vi "CalibBoard.vi"() -> ()   [LabVIEW 2014]
uses:
  <vilib>/userdefined/High Color/IMAQdx.ctl
  <vilib>/vision/Image Controls.llb/IMAQ Image.ctl
  Ctrl/CalibBoardAction.ctl
  <vilib>/Utility/miscctls.llb/LVPositionTypeDef.ctl
  Ctrl/ColorImg.ctl
  Control/RobotActionMode.ctl
  Global/PanelSetting.vi
  <vilib>/vision/driver/NI_Vision_Acquisition_Software.lvlib
panel:
  in  "SelectCalib":bool caption="點位校正功能開啟"
  out "UpCamTool 2":cluster{"CP-J1-X":sgl, "CP-J2-Y":sgl}={"CP-J1-X"=-0.14151, "CP-J2-Y"=-65.0295} caption="相機中心" {"CP-J2-Y" format="%.3g"; "CP-J1-X" format="%.3g"}
  out "UpCamTool":refnum<vi>
  in  "Session In":T1
  in  "Btn_BoardSave":bool
  in  "file path (use dialog)":path
  out "ActQ":refnum<queue>
  in  "CalibPts":cluster{"X":dbl, "Y":dbl, "Z":dbl, "U":dbl}[](array[cluster])
  out "BoardPts":cluster{dbl, dbl}[][](array[cluster])
  out "CalibPoint":cluster{dbl, dbl}[](array[cluster])
  out "Current PositionRef":refnum<vi>
  in  "Current Position":T2 caption="當前點位坐標" {"CP-J6-W" format="%.3g"; "CP-J5-V" format="%.3g"; "CP-J4-U" format="%.3g"; "CP-J3_Z" format="%.3g"; "CP-J2-Y" format="%.3g"; "CP-J1-X" format="%.3g"}
  in  "Image":T3
  out "Btn_ExistRef":refnum<vi>
  in  "Btn_Exist":bool=TRUE
  in  "Tab Control":enum32{"Set", "Data"}(tab)
  out "CirclesResult":T4(array[cluster]) caption="圓結果"
  in  "SetStartPoint":bool
  in  "PointArray":cluster{"X":i32, "Y":i32} caption="標準板陣列"
  in  "PointsDis":cluster{"DeltaX":dbl, "DeltaY":dbl} caption="點距離(mm)"
  in  "StartPoint":cluster{"X":dbl, "Y":dbl, "Z":dbl, "U":dbl} caption="起始點位"
  in  "StartCalib":bool
  in  "CalibBoardImg":T3(plugin-control)
  in  "Clu_BoardCircleParameter":T5={"Extraction Mode"=enum."Normal", "Edge Threshold"=40, "Edge Filter Size"=enum."Normal"} caption="搜尋參數"
  in  "Btn_SetROI":bool
  in  "Btn_BoardDetect":bool
  in  "Btn_BoardSnap":bool
  in  "Circle Descriptor":cluster{"Min Radius":dbl, "Max Radius":dbl}={"Min Radius"=30.0, "Max Radius"=100.0} caption="圓半徑"
  in  "ROI":T6
  out "Numbers":i32
  in  "Index":i32
  in  "CalibBoardData":string[][](table)
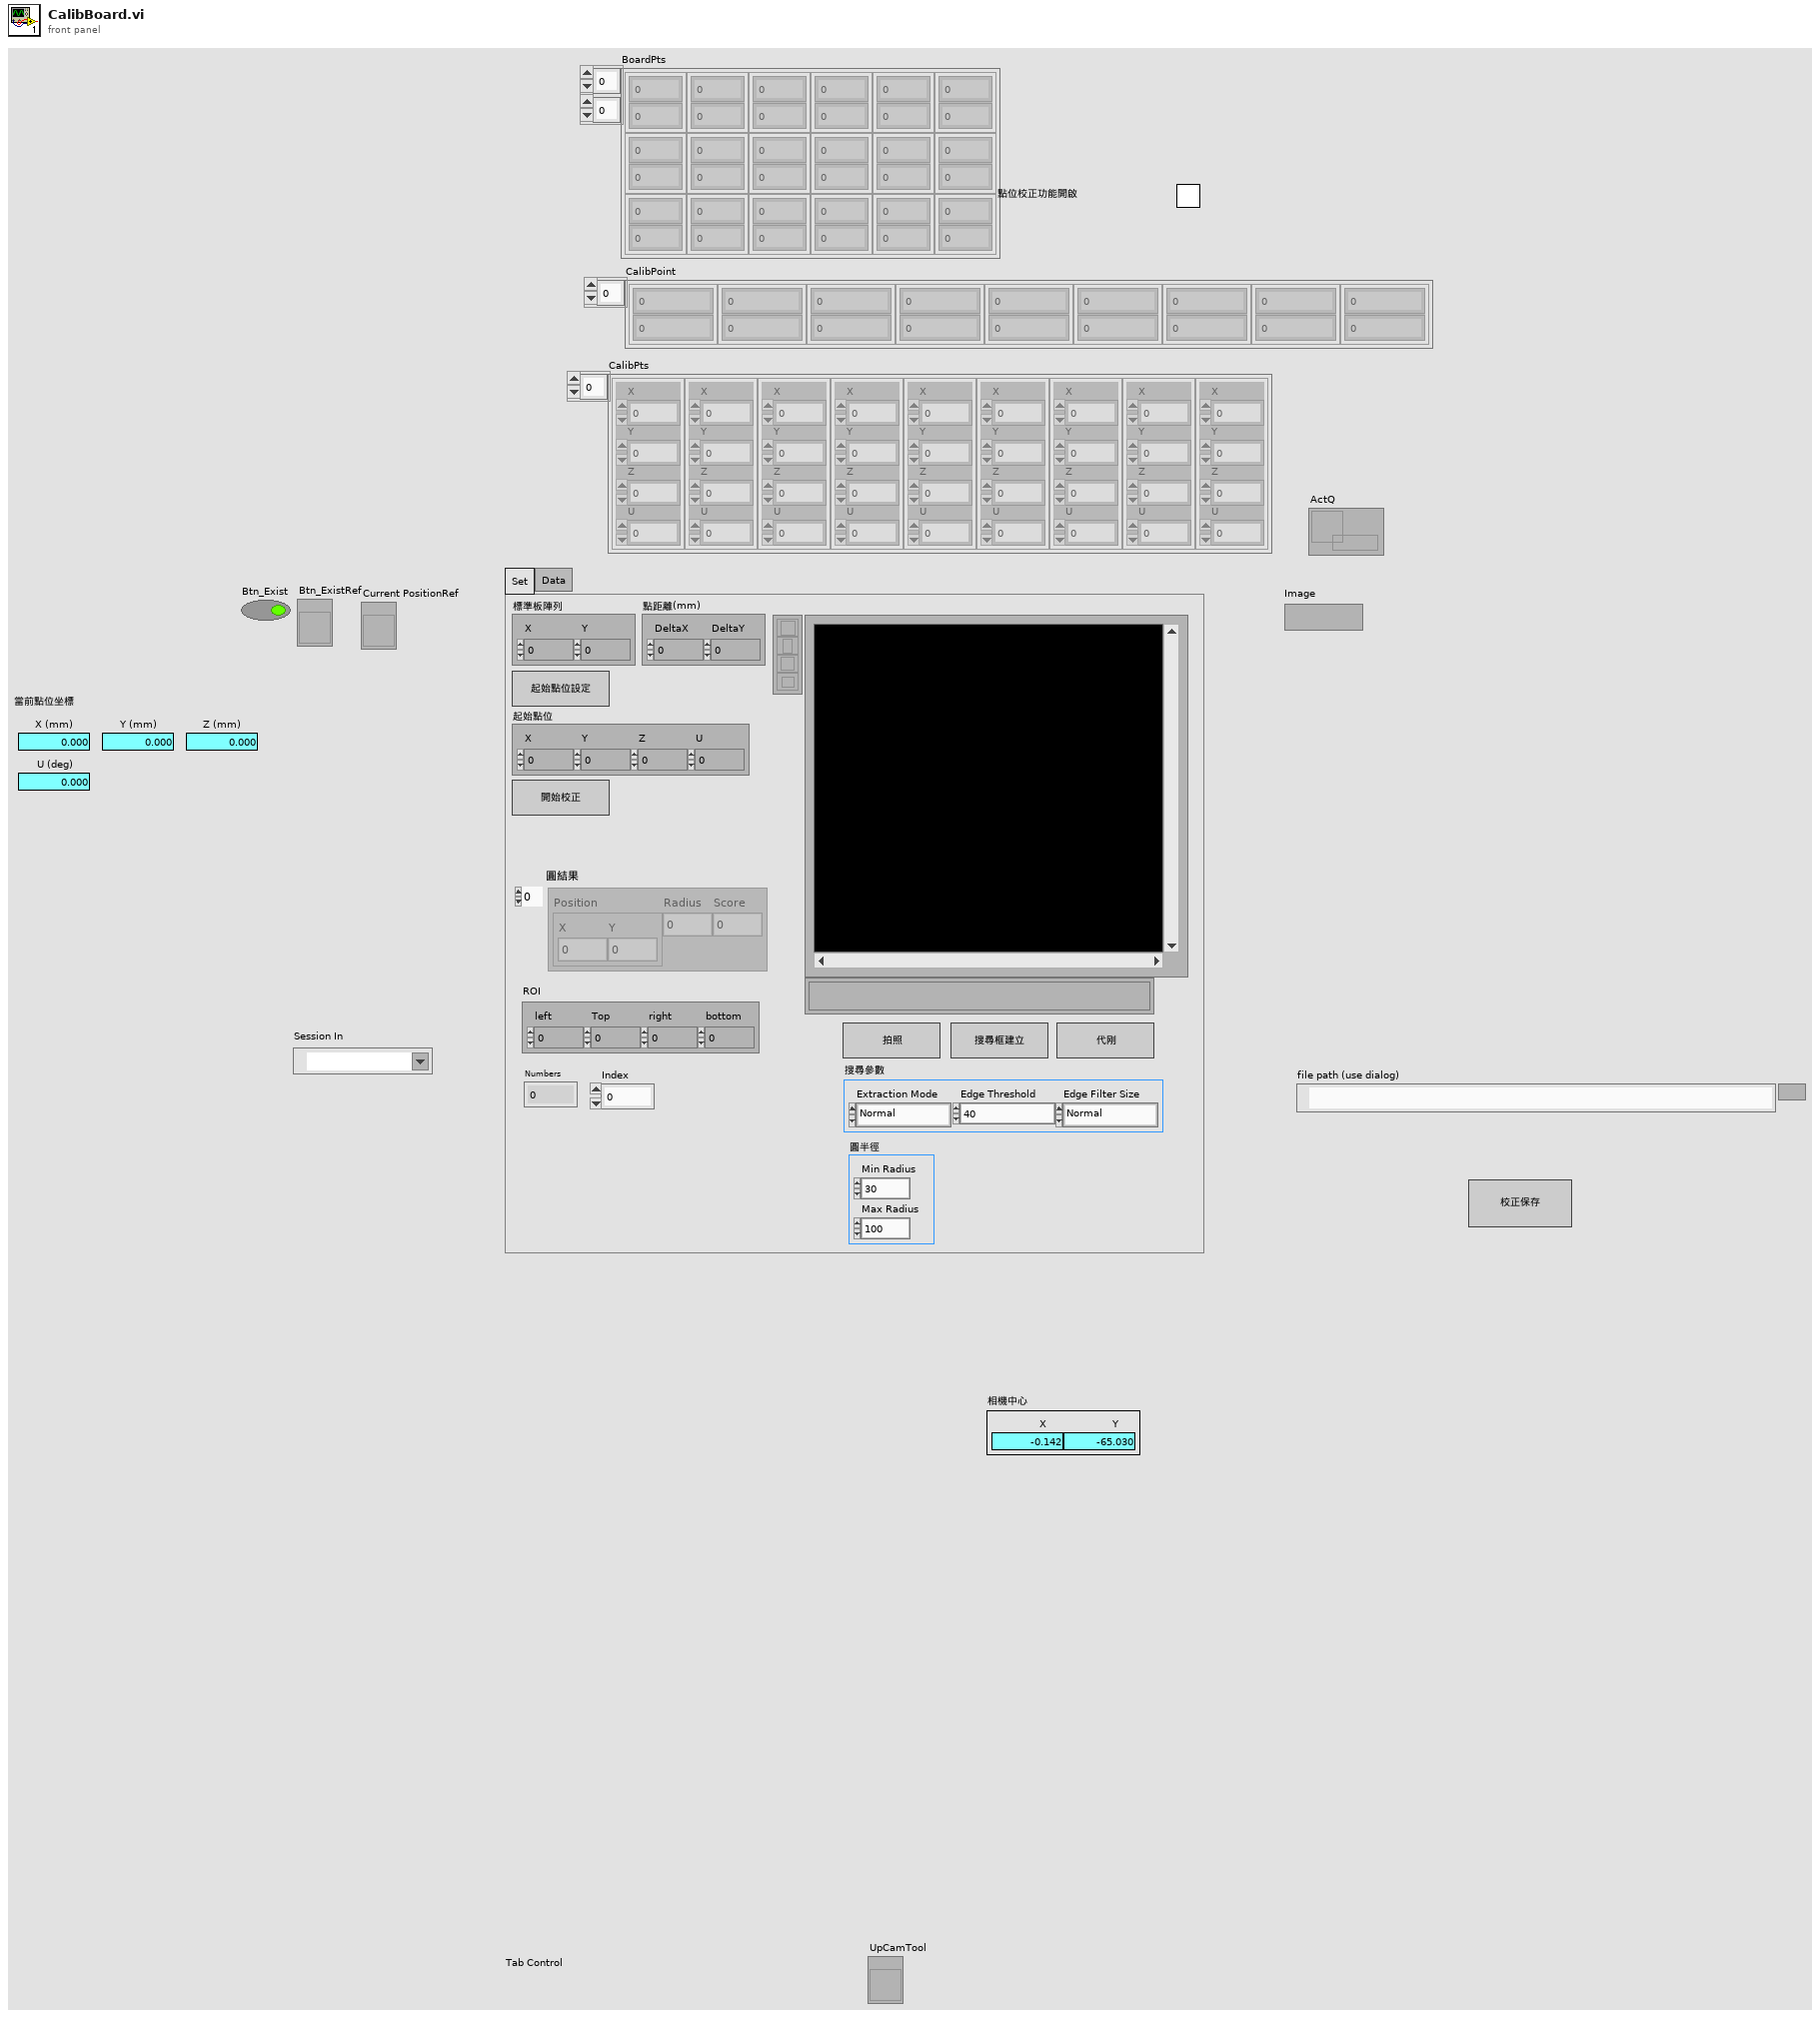
[diagram p1: front panel]
types:
  T1 = typedef "IMAQdx.ctl" = refnum<k21>
  T2 = cluster{"CP-J1-X":sgl, "CP-J2-Y":sgl, "CP-J3_Z":sgl, "CP-J4-U":sgl, "CP-J5-V":sgl, "CP-J6-W":sgl}
  T3 = typedef "IMAQ Image.ctl" = refnum<image>
  T4 = cluster{"Position":cluster{"X":sgl, "Y":sgl}, "Radius":dbl, "Score":dbl}[]
  T5 = cluster{"Extraction Mode":enum16{"Normal", "Uniform Regions"}, "Edge Threshold":i32, "Edge Filter Size":enum16{"Fine", "Normal"}}
  T6 = cluster{"left":i32, "Top":i32, "right":i32, "bottom":i32}
  T7 = enum16{"initialref", "save", "load", "UpDataToUI", "write", "read"}
  T8 = typedef "CalibBoardAction.ctl" = enum16{"CalibBoard", "Snap", "BoardCircleDectect", "CaculateOffset", "Exit"}
  T9 = typedef "RobotActionMode.ctl" = cluster{"PM_1":i32, "PM_2":i32}
  T10 = typedef "ColorImg.ctl" = enum16{"CBSource", "CBShow", "CBToProcess"}
  T11 = cluster{"Curve Parameters":cluster{"Extraction Mode":enum16{"Normal", "Uniform Regions"}, "Edge Threshold":i32, "Edge Filter Size":enum16{"Fine", "Normal"}, "Min Length":i32, "Row Search Step Size":i32, "Col Search Step Size":i32, "Max Endpoint Gap":i32, "Closed":bool, "Subpixel":bool}, "Circle Descriptor":cluster{"Min Radius":dbl, "Max Radius":dbl}, "Match Options":cluster{"Rotation":bool, "Scale":bool, "Occlusion":bool, "Range Settings":cluster{"Match Constraints":enum16{"Rotation Angle (degrees)", "Scale Factor (%)", "Occlusion (%)"}, "Min":dbl, "Max":dbl}[]}, "Minimum match score":dbl, "SetCircleNum":i32}
  T12 = typedef "LVPositionTypeDef.ctl" = cluster{"Left":i32, "Top":i32}
  T13 = cluster{"PointArray":refnum<vi>, "PointsDis":refnum<vi>, "StartPoint":refnum<vi>, "ROI":refnum<vi>, "Clu_BoardCircleParameter":refnum<vi>, "Circle Descriptor":refnum<vi>, "BoardPts":refnum<vi>, "CalibPoint":refnum<vi>, "CalibPts":refnum<vi>, "SelectCalib":refnum<vi>}
  T14 = cluster{"Global Rectangle":i32[], "Contours":cluster{"Contour Type":u32, "ROI Type":u32, "Points":i32[]}[]}
  T15 = typedef "IMAQ Rectangle" = cluster{"Left":i32, "Top":i32, "Right":i32, "Bottom":i32, "Rotation":dbl}
  T16 = cluster{"Left":i32, "Top":i32, "Right":i32, "Bottom":i32}
  T17 = cluster{"CP-J1-X":sgl, "CP-J2-Y":sgl, "CP-J3_Z":sgl, "CP-J4-U":sgl}
  T18 = cluster{"left":i32, "Top":i32, "right":i32, "bottom":i32, dbl}
  T19 = typedef "ROI Descriptor" = cluster{"Global Rectangle":i32[], "Contours":cluster{"ID":enum32{"External", "Internal"}, "Type":u32, "Coordinates":i32[]}[]}
  T20 = cluster{"Position":cluster{"X":sgl, "Y":sgl}, "Radius":dbl, "Score":dbl}
  T21 = cluster{"[0]":sgl, "[1]":sgl, "[2]":sgl, "[3]":sgl}
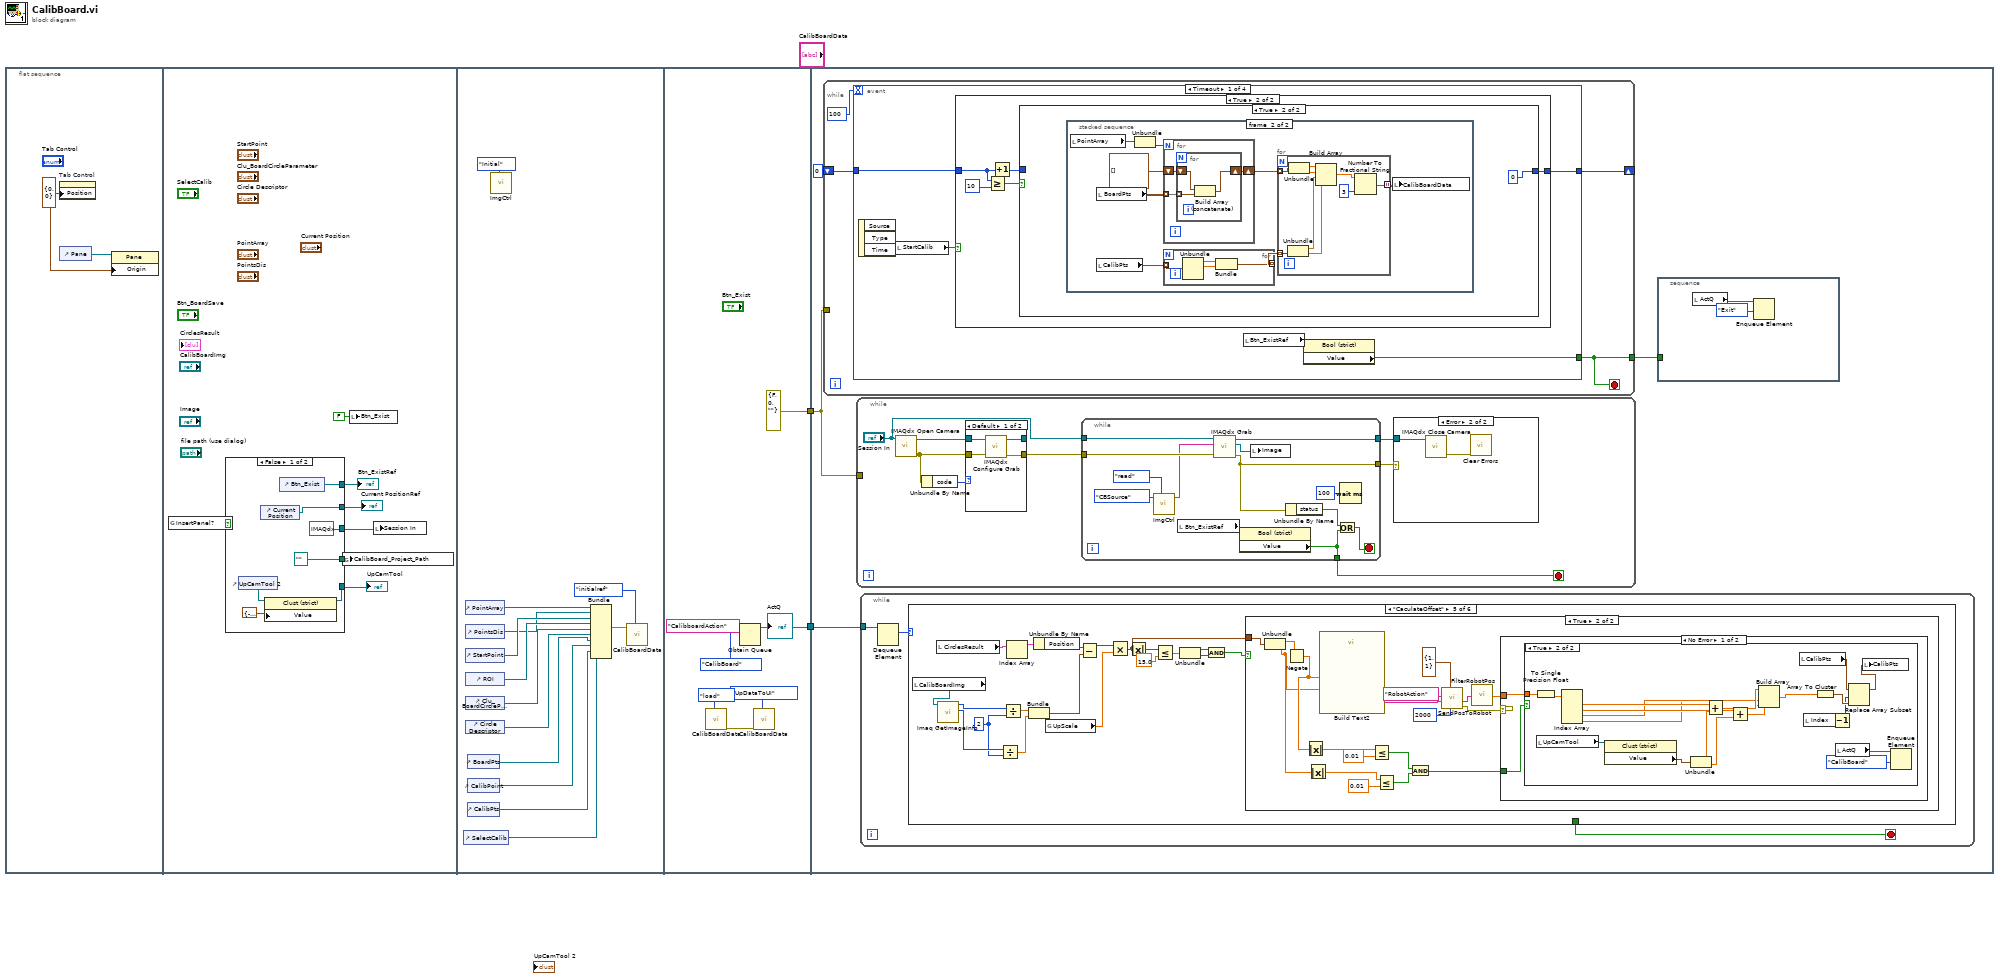
[diagram p0: block diagram]
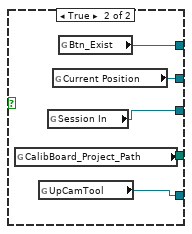
[diagram p2: hidden frame]
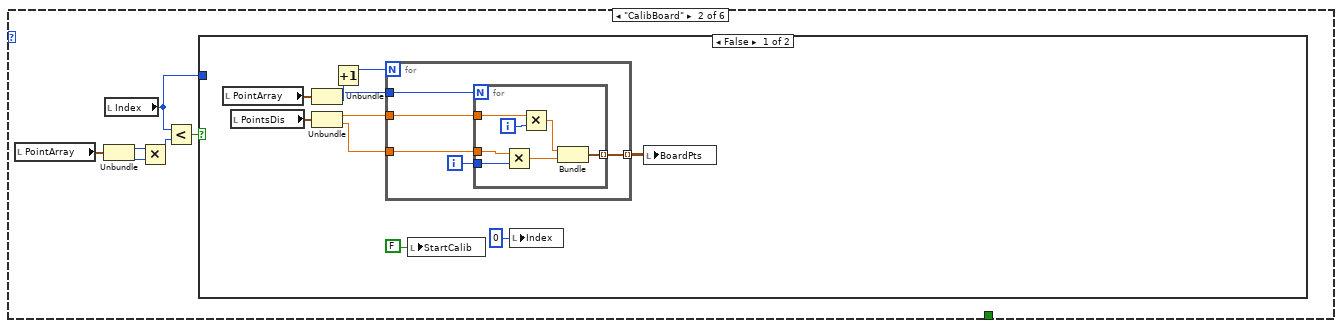
[diagram p4: hidden frame]
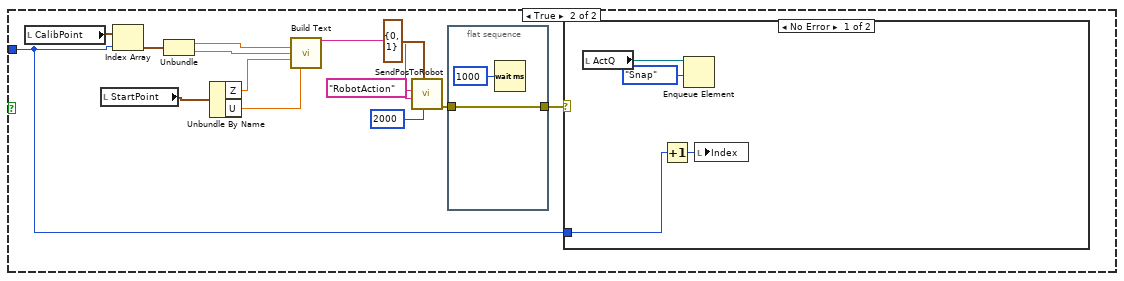
[diagram p5: hidden frame]
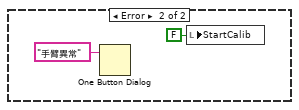
[diagram p6: hidden frame]
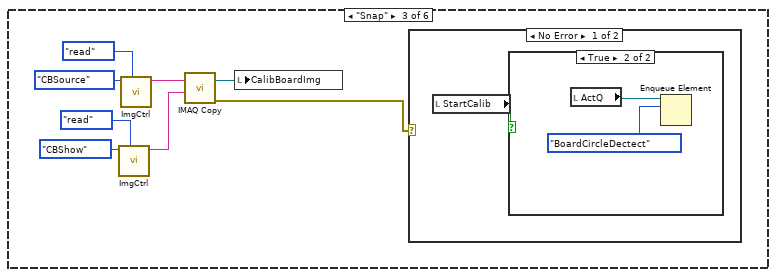
[diagram p7: hidden frame]
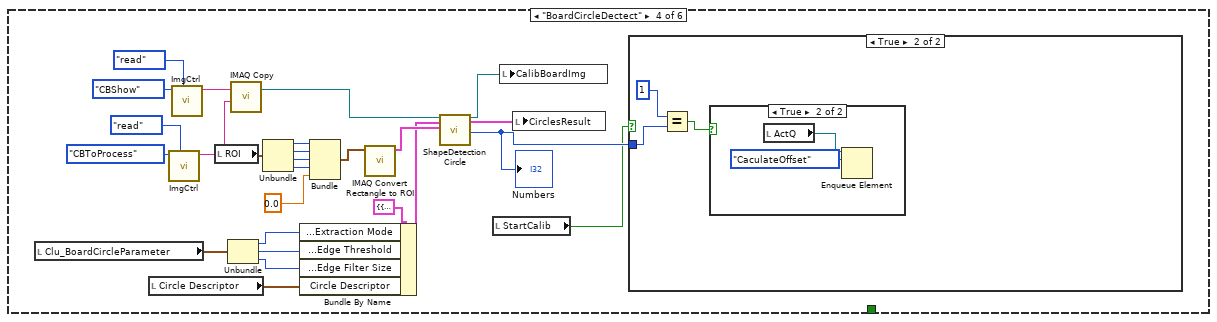
[diagram p10: hidden frame]
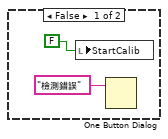
[diagram p12: hidden frame]
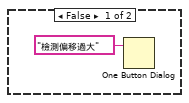
[diagram p13: hidden frame]
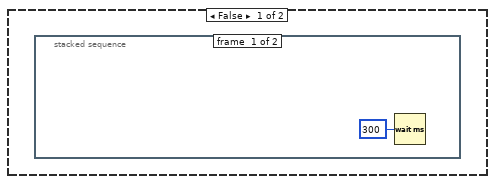
[diagram p14: hidden frame]
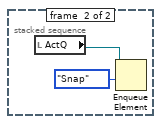
[diagram p15: hidden frame]
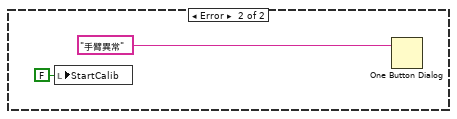
[diagram p16: hidden frame]
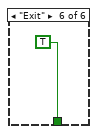
[diagram p17: hidden frame]
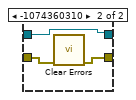
[diagram p18: hidden frame]
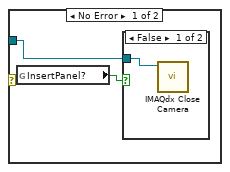
[diagram p19: hidden frame]
diagram:
  n1 = flat-sequence {
    tunnel: [errorcluster {"status"=FALSE, "code"=0, "source"=""} ("error constant")] -> w2
    tunnel: [w40] -> w1
    tunnel: w2 -> [w47]
    tunnel: w1 -> [w46]
    frame #0 {
      w3 = T12 {"Left"=0, "Top"=0} ("Position")
      n2 = property on="Tab Control" class="TabCtl (strict)"("Position"=w3) -> ()  [unwired: 2 in, 2 out]
      n3 = control-ref of="Pane"() -> (w4:refnum<vi>)
      n4 = property class="Pane"(reference=w4, "Origin"=w3) -> ()  [unwired: 1 in, 2 out]
    }
    frame #1 {
      n5 = global read "PanelSetting.vi" "InsertPanel?"() -> (w11:bool)
      n6 = case shown="False" w11 {
        tunnel: [w18 w23] -> w10
        tunnel: [w17 w22] -> w9
        tunnel: [T1 refnum ("Session In") w21] -> w8
        tunnel: [path "" ("Project_Path") w20] -> w6
        tunnel: [w12 w19] -> w5
        frame False {
          n7 = control-ref of="UpCamTool 2"() -> (w14:refnum<vi>)
          n8 = control-ref of="Current Position"() -> (w17:refnum<vi>)
          n9 = property class="Clust (strict)"(reference=w14, "Value"=cluster{"CP-J1-X":sgl, "CP-J2-Y":sgl} {"CP-J1-X"=-0.142, "CP-J2-Y"=-65.03}) -> (reference out=w12:refnum<vi>)  [unwired: 1 in, 1 out]
          n10 = control-ref of="Btn_Exist"() -> (w18:refnum<vi>)
        }
        frame True {
          n11 = global read "PanelSetting.vi" "CalibBoard_Project_Path"() -> (w20:path)
          n12 = global read "PanelSetting.vi" "UpCamTool"() -> (w19:refnum<vi>)
          n13 = global read "PanelSetting.vi" "Session In"() -> (w21:T1)
          n14 = global read "PanelSetting.vi" "Current Position"() -> (w22:refnum<vi>)
          n15 = global read "PanelSetting.vi" "Btn_Exist"() -> (w23:refnum<vi>)
        }
      }
      "Btn_ExistRef" <- w10
      "Current PositionRef" <- w9
      "UpCamTool" <- w5
      n16 = global write "PanelSetting.vi" "CalibBoard_Project_Path"(w6) -> ()
      n17 = local write "Btn_Exist"(FALSE ("Btn_Exist")) -> ()
      n18 = local write "Session In"(w8) -> ()
    }
    frame #2 {
      n19 = control-ref of="SelectCalib"() -> (w24:refnum<vi>)
      n20 = control-ref of="PointArray"() -> (w27:refnum<vi>)
      n21 = control-ref of="PointsDis"() -> (w28:refnum<vi>)
      n22 = control-ref of="StartPoint"() -> (w29:refnum<vi>)
      n23 = control-ref of="ROI"() -> (w30:refnum<vi>)
      n24 = control-ref of="Clu_BoardCircleParameter"() -> (w31:refnum<vi>)
      n25 = control-ref of="Circle Descriptor"() -> (w32:refnum<vi>)
      n26 = control-ref of="BoardPts"() -> (w33:refnum<vi>)
      n27 = control-ref of="CalibPoint"() -> (w34:refnum<vi>)
      n28 = control-ref of="CalibPts"() -> (w35:refnum<vi>)
      n29 = call "ImgCtrl.vi"("Action"=enum16{"Initial", "read", "release"}."Initial") -> ()  [unwired: 9 in, 2 out]
      n30 = Bundle("PointArray"=w27, "PointsDis"=w28, "StartPoint"=w29, "ROI"=w30, "Clu_BoardCircleParameter"=w31, "Circle Descriptor"=w32, "BoardPts"=w33, "CalibPoint"=w34, "CalibPts"=w35, "SelectCalib"=w24) -> (w26:T13)  [unwired: 1 in]
      n31 = call "CalibBoardData.vi"("Enum"=T7."initialref", "RefIn"=w26) -> ()  [unwired: 8 in, 2 out]
    }
    frame #3 {
      n32 = call "CalibBoardData.vi"("Enum"=T7."load") -> ("error out"=w37:errorcluster)  [unwired: 9 in, 1 out]
      n33 = Obtain Queue(name (unnamed)="CalibboardAction", element data type=CalibBoardAction."CalibBoard") -> (queue out=w40:refnum<queue>)  [unwired: 3 in, 2 out]
      "ActQ" <- w40
      n34 = call "CalibBoardData.vi"("Enum"=T7."UpDataToUI", "error in"=w37) -> ()  [unwired: 8 in, 2 out]
    }
    frame #4 {
      n35 = while {
        tunnel: w47 -> [_]
        tunnel: [w248] -> w45
        shift-right: [w246] -> _
        shift-left: 0 -> [w247]
        stop <- w248 stop-if-true
        n36 = event shown="[0] Timeout" {
          selector: _ -> [_ _ _ _]
          dyn-events: _ -> [_ _ _ _]
          timeout: 100 -> [_ _ _ _]
          tunnel: [w254 _ _ _] -> w248
          tunnel: w247 -> [w251 _ _ _]
          tunnel: [w250 _ _ _] -> w246
          event Timeout {
            n37 = event-data() -> ()  [unwired: 1 in, 3 out]
            n38 = local read "StartCalib"() -> (w252:bool)
            n39 = case shown="True" w252 {
              tunnel: w251 -> [w255 w257]
              tunnel: [w255 w258] -> w250
              frame False {
              }
              frame True {
                n40 = Greater Or Equal?(x=w257, y=10) -> (x >= y?=w259:bool)
                n41 = Increment(x=w257) -> (x+1=w256:i32)
                n42 = case shown="True" w259 {
                  tunnel: [w261 0] -> w258
                  tunnel: w256 -> [w261 _]
                  frame False {
                  }
                  frame True {
                    n43 = stacked-sequence {
                      frame #0 {
                        n44 = local read "PointArray"() -> (w267:cluster{"X":i32, "Y":i32})
                        n45 = Unbundle(w267) -> ("X"=w265:i32, "Y"=w266:i32)
                        n46 = Multiply(x=w265, y=w266) -> (x*y=w264:i32)
                        n47 = for {
                          N: w264 -> [_]
                          tunnel: [w271] -> w263 mode=indexing
                          i -> [w272]
                          n48 = Number To Decimal String(number=w272) -> (decimal integer string=w271:string)  [unwired: 1 in]
                        }
                        n49 = Initialize Array("4", 0 ("dimension size"), w264) -> (w270:string[][])
                        n50 = local write "CalibBoardData"(w270) -> ()
                        n51 = property on="CalibBoardData" class="Tbl (strict)"("Row Headers[]"=w263) -> ()  [unwired: 2 in, 2 out]
                      }
                      frame #1 {
                        n52 = local read "PointArray"() -> (w274:cluster{"X":i32, "Y":i32})
                        n53 = local read "CalibPts"() -> (w278:cluster{"X":dbl, "Y":dbl, "Z":dbl, "U":dbl}[])
                        n54 = local read "BoardPts"() -> (w276:cluster{dbl, dbl}[][])
                        n55 = Unbundle(w274) -> ("Y"=w273:i32)  [unwired: 1 out]
                        n56 = for {
                          N: w273 -> [_]
                          tunnel: w276 -> [w296] mode=indexing
                          shift-right: [w294] -> w280
                          shift-left: cluster{dbl, dbl}[] [] -> [w295]
                          n57 = for {
                            tunnel: w296 -> [w299] mode=indexing
                            shift-right: [w297] -> w294
                            shift-left: w295 -> [w298]
                            n58 = Build Array (concatenate)(w298, w299) -> (w297:cluster{dbl, dbl}[])
                          }
                        }
                        n59 = for {
                          tunnel: w278 -> [w293] mode=indexing
                          tunnel: [w290] -> w279 mode=indexing
                          n60 = Unbundle(w293) -> ("X"=w291:dbl, "Y"=w292:dbl)  [unwired: 2 out]
                          n61 = Bundle("X"=w291, "Y"=w292) -> (w290:cluster{"X":dbl, "Y":dbl})  [unwired: 1 in]
                        }
                        n62 = for {
                          tunnel: w279 -> [w288] mode=indexing
                          tunnel: w280 -> [w289] mode=indexing
                          tunnel: [w281] -> w275 mode=indexing
                          n63 = Unbundle(w288) -> ("X"=w285:dbl, "Y"=w284:dbl)
                          n64 = Unbundle(w289) -> (w287:dbl, w286:dbl)
                          n65 = Build Array(w287, w286, w285, w284) -> (w283:dbl[])
                          n66 = Number To Fractional String(number=w283, precision (6)=i16 3) -> (F-format string=w281:string[])  [unwired: 2 in]
                        }
                        n67 = local write "CalibBoardData"(w275) -> ()
                      }
                    }
                  }
                }
              }
            }
            n68 = local read "Btn_ExistRef"() -> (w253:refnum<vi>)
            n69 = property class="Bool (strict)"(reference=w253) -> ("Value"=w254:bool)  [unwired: 1 in, 2 out]
          }
          event "Btn_BoardSnap", "Btn_SetROI", "Btn_BoardDetect", "SetStartPoint": Value Change {
            n70 = event-data() -> ("CtlRef"=w302:refnum<vi>)  [unwired: 1 in, 5 out]
            n71 = property class="Bool"(reference=w302) -> ("Label.Text"=w301:string)  [unwired: 1 in, 2 out]
            n72 = local read "ActQ"() -> (w300:refnum<queue>)
            n73 = case shown="\"SetStartPoint\"" w301 {
              tunnel: w300 -> [_ w303 _ w313 _]
              frame "False", Default {
              }
              frame "Btn_BoardSnap" {
                n74 = Enqueue Element(queue=w303, element=CalibBoardAction."Snap") -> ()  [unwired: 2 in, 3 out]
              }
              frame "Btn_SetROI" {
                n75 = property on="CalibBoardImg" class="ImageControl"() -> ("ROI"=w311:T14)  [unwired: 2 in, 2 out]
                n76 = call "IMAQ Convert ROI to Rectangle"("ROI Descriptor"=w311) -> ("Rectangle"=w310:T15)  [unwired: 8 in, 1 out]
                n77 = Unbundle(w310) -> ("Left"=w309:i32, "Top"=w308:i32, "Right"=w306:i32, "Bottom"=w307:i32)  [unwired: 1 out]
                n78 = Bundle("Left"=w309, "Top"=w308, "Right"=w306, "Bottom"=w307) -> (w305:T16)  [unwired: 1 in]
                n79 = local write "ROI"(w305) -> ()
              }
              frame "Btn_BoardDetect" {
                n80 = Enqueue Element(queue=w313, element=CalibBoardAction."BoardCircleDectect") -> ()  [unwired: 2 in, 3 out]
              }
              frame "SetStartPoint" {
                n81 = local read "Current PositionRef"() -> (w320:refnum<vi>)
                n82 = property class="Clust (strict)"(reference=w320) -> ("Value"=w319:T2)  [unwired: 1 in, 2 out]
                n83 = Unbundle(w319) -> ("CP-J1-X"=w318:sgl, "CP-J2-Y"=w317:sgl, "CP-J3_Z"=w316:sgl, "CP-J4-U"=w315:sgl)  [unwired: 2 out]
                n84 = Bundle("CP-J1-X"=w318, "CP-J2-Y"=w317, "CP-J3_Z"=w316, "CP-J4-U"=w315) -> (w314:T17)  [unwired: 1 in]
                n85 = local write "StartPoint"(w314) -> ()
              }
            }
          }
          event "StartCalib": Value Change {
            n86 = event-data() -> ("NewVal"=w321:bool)  [unwired: 1 in, 5 out]
            n87 = case shown="True" w321 {
              frame False {
              }
              frame True {
                n88 = stacked-sequence {
                  frame #0 {
                    n89 = local read "PointArray"() -> (w328:cluster{"X":i32, "Y":i32})
                    n90 = local read "PointsDis"() -> (w329:cluster{"DeltaX":dbl, "DeltaY":dbl})
                    n91 = Unbundle(w328) -> ("X"=w326:i32, "Y"=w327:i32)
                    n92 = Unbundle(w329) -> ("DeltaX"=w325:dbl, "DeltaY"=w324:dbl)
                    n93 = Increment(x=w327) -> (x+1=w322:i32)
                    n94 = for {
                      N: w322 -> [_]
                      tunnel: w326 -> [w337]
                      tunnel: w325 -> [w336]
                      tunnel: w324 -> [w334]
                      shift-right: [w332] -> w330
                      shift-left: cluster{dbl, dbl}[] [] -> [w331]
                      i -> [w335]
                      n95 = for {
                        N: w337 -> [_]
                        tunnel: w336 -> [w349]
                        tunnel: w335 -> [w344]
                        tunnel: w334 -> [w343]
                        tunnel: [w339] -> w333 mode=indexing
                        i -> [w348]
                        n96 = local read "StartPoint"() -> (w338:cluster{"X":dbl, "Y":dbl, "Z":dbl, "U":dbl})
                        n97 = Multiply(x=w343, y=w344) -> (x*y=w345:dbl)
                        n98 = Unbundle(w338) -> ("X"=w346:dbl, "Y"=w342:dbl)  [unwired: 2 out]
                        n99 = Multiply(x=w349, y=w348) -> (x*y=w347:dbl)
                        n100 = Add(x=w346, y=w347) -> (x+y=w341:dbl)
                        n101 = Add(x=w342, y=w345) -> (x+y=w340:dbl)
                        n102 = Bundle(w341, w340) -> (w339:cluster{dbl, dbl})  [unwired: 1 in]
                      }
                      n103 = Build Array (concatenate)(w331, w333) -> (w332:cluster{dbl, dbl}[])
                    }
                    "CalibPoint" <- w330
                  }
                  frame #1 {
                    n104 = local read "PointArray"() -> (w356:cluster{"X":i32, "Y":i32})
                    n105 = local read "PointsDis"() -> (w355:cluster{"DeltaX":dbl, "DeltaY":dbl})
                    n106 = Unbundle(w356) -> ("X"=w353:i32, "Y"=w352:i32)
                    n107 = Unbundle(w355) -> ("DeltaX"=w354:dbl, "DeltaY"=w351:dbl)
                    n108 = Increment(x=w352) -> (x+1=w350:i32)
                    n109 = for {
                      N: w350 -> [_]
                      tunnel: w353 -> [w362]
                      tunnel: w354 -> [w361]
                      tunnel: w351 -> [w360]
                      tunnel: [w358] -> w357 mode=indexing
                      i -> [w359]
                      n110 = for {
                        N: w362 -> [_]
                        tunnel: w361 -> [w368]
                        tunnel: w360 -> [w367]
                        tunnel: w359 -> [w366]
                        tunnel: [w363] -> w358 mode=indexing
                        i -> [w369]
                        n111 = Multiply(x=w367, y=w366) -> (x*y=w364:dbl)
                        n112 = Multiply(x=w368, y=w369) -> (x*y=w365:dbl)
                        n113 = Bundle(w365, w364) -> (w363:cluster{dbl, dbl})  [unwired: 1 in]
                      }
                    }
                    "BoardPts" <- w357
                  }
                  frame #2 {
                    n114 = call "Prompt User for Input"() -> ("Index"=w375:dbl, "OK"=w376:bool)  [unwired: 17 in, 1 out]
                    n115 = local read "PointArray"() -> (w374:cluster{"X":i32, "Y":i32})
                    n116 = Unbundle(w374) -> ("X"=w371:i32, "Y"=w373:i32)
                    n117 = Increment(x=w373) -> (x+1=w372:i32)
                    n118 = Multiply(x=w371, y=w372) -> (x*y=w370:i32)
                    n119 = case shown="False" w376 {
                      tunnel: w375 -> [_ w377]
                      tunnel: w370 -> [_ w378]
                      frame False {
                      }
                      frame True {
                        n120 = local write "Index"(w377) -> ()
                        n121 = Equal To 0?(x=w377) -> (x = 0?=w379:bool)
                        n122 = case shown="True" w379 {
                          tunnel: w377 -> [_ _]
                          tunnel: w378 -> [_ w380]
                          frame False {
                          }
                          frame True {
                            n123 = Initialize Array(cluster{"X":sgl, "Y":sgl, "Z":sgl, "U":sgl} {"X"=0.0, "Y"=0.0, "Z"=0.0, "U"=0.0} ("cluster"), w380) -> (w381:cluster{"X":sgl, "Y":sgl, "Z":sgl, "U":sgl}[])
                            n124 = local write "CalibPts"(w381) -> ()
                          }
                        }
                      }
                    }
                  }
                  frame #3 {
                    n125 = local read "ActQ"() -> (w383:refnum<queue>)
                    n126 = Enqueue Element(queue=w383, element=CalibBoardAction."CalibBoard") -> ()  [unwired: 2 in, 3 out]
                  }
                }
              }
            }
          }
          event "Tab Control": Value Change {
            n127 = event-data() -> ("NewVal"=w385:enum32{"Set", "Data"})  [unwired: 1 in, 5 out]
            n128 = case shown="\"Data\"" w385 {
              frame "Set", Default {
              }
              frame "Data" {
                n129 = stacked-sequence {
                  frame #0 {
                    n130 = local read "PointArray"() -> (w390:cluster{"X":i32, "Y":i32})
                    n131 = Unbundle(w390) -> ("X"=w388:i32, "Y"=w389:i32)
                    n132 = Multiply(x=w388, y=w389) -> (x*y=w387:i32)
                    n133 = Initialize Array("4", 0 ("dimension size"), w387) -> (w393:string[][])
                    n134 = for {
                      N: w387 -> [_]
                      tunnel: [w394] -> w386 mode=indexing
                      i -> [w395]
                      n135 = Number To Decimal String(number=w395) -> (decimal integer string=w394:string)  [unwired: 1 in]
                    }
                    n136 = local write "CalibBoardData"(w393) -> ()
                    n137 = property on="CalibBoardData" class="Tbl (strict)"("Row Headers[]"=w386) -> ()  [unwired: 2 in, 2 out]
                  }
                  frame #1 {
                    n138 = local read "PointArray"() -> (w397:cluster{"X":i32, "Y":i32})
                    n139 = local read "CalibPts"() -> (w401:cluster{"X":dbl, "Y":dbl, "Z":dbl, "U":dbl}[])
                    n140 = local read "BoardPts"() -> (w399:cluster{dbl, dbl}[][])
                    n141 = Unbundle(w397) -> ("Y"=w396:i32)  [unwired: 1 out]
                    n142 = for {
                      N: w396 -> [_]
                      tunnel: w399 -> [w419] mode=indexing
                      shift-right: [w417] -> w403
                      shift-left: cluster{dbl, dbl}[] [] -> [w418]
                      n143 = for {
                        tunnel: w419 -> [w422] mode=indexing
                        shift-right: [w420] -> w417
                        shift-left: w418 -> [w421]
                        n144 = Build Array (concatenate)(w421, w422) -> (w420:cluster{dbl, dbl}[])
                      }
                    }
                    n145 = for {
                      tunnel: w401 -> [w416] mode=indexing
                      tunnel: [w413] -> w402 mode=indexing
                      n146 = Unbundle(w416) -> ("X"=w414:dbl, "Y"=w415:dbl)  [unwired: 2 out]
                      n147 = Bundle("X"=w414, "Y"=w415) -> (w413:cluster{"X":dbl, "Y":dbl})  [unwired: 1 in]
                    }
                    n148 = for {
                      tunnel: w402 -> [w411] mode=indexing
                      tunnel: w403 -> [w412] mode=indexing
                      tunnel: [w404] -> w398 mode=indexing
                      n149 = Unbundle(w411) -> ("X"=w408:dbl, "Y"=w407:dbl)
                      n150 = Unbundle(w412) -> (w410:dbl, w409:dbl)
                      n151 = Build Array(w410, w409, w408, w407) -> (w406:dbl[])
                      n152 = Number To Fractional String(number=w406, precision (6)=i16 3) -> (F-format string=w404:string[])  [unwired: 2 in]
                    }
                    n153 = local write "CalibBoardData"(w398) -> ()
                  }
                }
              }
            }
          }
        }
      }
      n154 = while {
        tunnel: w47 -> [_]
        stop <- w220 stop-if-true
        n155 = call <vilib>:"IMAQdx Open Camera.vi"("Session In"="Session In") -> ("error out"=w216:errorcluster, "Session Out"=w214:T1)  [unwired: 9 in]
        n156 = Unbundle By Name(w216) -> ("code"=w217:i32)
        n157 = case shown="Default" w217 {
          tunnel: w216 -> [w221 w227]
          tunnel: [w223 w226] -> w215
          tunnel: [w224 w225] -> _
          tunnel: w214 -> [w222 w225]
          frame Default {
            n158 = call <vilib>:"IMAQdx Configure Grab.vi"("error in"=w221, "Session In"=w222) -> ("error out"=w223:errorcluster, "Session Out"=w224:T1)  [unwired: 8 in]
          }
          frame -1074360310 {
            n159 = call <vilib>:"Clear Errors.vi"("error in (no error)"=w227) -> ("error out"=w226:errorcluster)  [unwired: 5 in, 1 out]
          }
        }
        n160 = while {
          tunnel: "Session In" -> [w245]
          tunnel: w215 -> [w244]
          tunnel: [w237] -> w220
          tunnel: [w236] -> w218
          tunnel: [w235] -> w219
          stop <- w238 stop-if-true
          n161 = call "ImgCtrl.vi"("Action"=enum16{"Initial", "read", "release"}."read", "ColorImg"=ColorImg."CBSource") -> ("ColorImg"=w241:string)  [unwired: 8 in, 1 out]
          n162 = local read "Btn_ExistRef"() -> (w233:refnum<vi>)
          n163 = call <vilib>:"IMAQdx Grab.vi"("error in"=w244, "Image In"=w241, "Session In"=w245) -> ("error out"=w235:errorcluster, "Image Out"=w240:T3, "Session Out"=w236:T1)  [unwired: 5 in, 1 out]
          n164 = property class="Bool (strict)"(reference=w233) -> ("Value"=w237:bool)  [unwired: 1 in, 2 out]
          n165 = local write "Image"(w240) -> ()
          n166 = Unbundle By Name(w235) -> ("status"=w239:bool)
          n167 = Or(x=w239, y=w237) -> (x .or. y?=w238:bool)
          n168 = Wait (ms)(milliseconds to wait=u32 100) -> ()  [unwired: 1 out]
        }
        n169 = case shown="Error" w219 {
          tunnel: w218 -> [w228 w232]
          frame No Error {
            n170 = global read "PanelSetting.vi" "InsertPanel?"() -> (w229:bool)
            n171 = case shown="False" w229 {
              tunnel: w228 -> [w230 _]
              frame False {
                n172 = call <vilib>:"IMAQdx Close Camera.vi"("Session In"=w230) -> ()  [unwired: 10 in, 1 out]
              }
              frame True {
              }
            }
          }
          frame Error {
            n173 = call <vilib>:"IMAQdx Close Camera.vi"("Session In"=w232) -> ("error out"=w231:errorcluster)  [unwired: 10 in]
            n174 = call <vilib>:"Clear Errors.vi"("error in (no error)"=w231) -> ()  [unwired: 5 in, 2 out]
          }
        }
      }
      n175 = while {
        tunnel: w46 -> [w52]
        stop <- w50 stop-if-true
        n176 = Dequeue Element(queue=w52) -> (element=w51:T8)  [unwired: 2 in, 3 out]
        n177 = case shown="\"CaculateOffset\"" w51 {
          tunnel: [_ _ _ _ _ TRUE] -> w50
          frame Default {
          }
          frame "CalibBoard" {
            n178 = local read "PointArray"() -> (w58:cluster{"X":i32, "Y":i32})
            n179 = Unbundle(w58) -> ("X"=w57:i32, "Y"=w56:i32)
            n180 = local read "Index"() -> (w53:i32)
            n181 = Multiply(x=w57, y=w56) -> (x*y=w55:i32)
            n182 = Less?(x=w53, y=w55) -> (x < y?=w54:bool)
            n183 = case shown="False" w54 {
              tunnel: w53 -> [_ w81]
              frame False {
                n184 = local read "PointArray"() -> (w62:cluster{"X":i32, "Y":i32})
                n185 = local read "PointsDis"() -> (w63:cluster{"DeltaX":dbl, "DeltaY":dbl})
                n186 = Unbundle(w62) -> ("X"=w65:i32, "Y"=w66:i32)
                n187 = Unbundle(w63) -> ("DeltaX"=w64:dbl, "DeltaY"=w67:dbl)
                n188 = Increment(x=w66) -> (x+1=w59:i32)
                n189 = for {
                  N: w59 -> [_]
                  tunnel: w65 -> [w73]
                  tunnel: w64 -> [w72]
                  tunnel: w67 -> [w71]
                  tunnel: [w69] -> w61 mode=indexing
                  i -> [w70]
                  n190 = for {
                    N: w73 -> [_]
                    tunnel: w72 -> [w79]
                    tunnel: w71 -> [w78]
                    tunnel: w70 -> [w77]
                    tunnel: [w74] -> w69 mode=indexing
                    i -> [w80]
                    n191 = Multiply(x=w78, y=w77) -> (x*y=w75:dbl)
                    n192 = Multiply(x=w79, y=w80) -> (x*y=w76:dbl)
                    n193 = Bundle(w76, w75) -> (w74:cluster{dbl, dbl})  [unwired: 1 in]
                  }
                }
                n194 = local write "StartCalib"(FALSE ("StartCalib")) -> ()
                n195 = local write "Index"(0 ("Index")) -> ()
                n196 = local write "BoardPts"(w61) -> ()
              }
              frame True {
                n197 = local read "CalibPoint"() -> (w94:cluster{dbl, dbl}[])
                n198 = local read "StartPoint"() -> (w92:cluster{"X":dbl, "Y":dbl, "Z":dbl, "U":dbl})
                n199 = Index Array(array=w94, index=w81) -> (element=w93:cluster{dbl, dbl})
                n200 = Unbundle(w93) -> (w91:dbl, w90:dbl)
                n201 = Unbundle By Name(w92) -> ("Z"=w89:dbl, "U"=w88:dbl)
                n202 = call "Build Text"("U"=w88, "X"=w91, "Y"=w90, "Z"=w89) -> ("Result"=w85:string)  [unwired: 10 in, 1 out]
                n203 = call "SendPosToRobot.vi"("Timeout(ms)"=u32 2000, "PM"=T9 {"PM_1"=0, "PM_2"=1}, "Position"=w85, "RobotCmd"="RobotAction") -> ("error out"=w83:errorcluster)  [unwired: 4 in, 3 out]
                n204 = flat-sequence {
                  tunnel: w83 -> [w101]
                  tunnel: [w101] -> w82
                  frame #0 {
                    n205 = Wait (ms)(milliseconds to wait=u32 1000) -> ()  [unwired: 1 out]
                  }
                }
                n206 = case shown="No Error" w82 {
                  tunnel: w81 -> [w95 _]
                  frame No Error {
                    n207 = local read "ActQ"() -> (w98:refnum<queue>)
                    n208 = Increment(x=w95) -> (x+1=w96:i32)
                    n209 = Enqueue Element(queue=w98, element=CalibBoardAction."Snap") -> ()  [unwired: 2 in, 3 out]
                    n210 = local write "Index"(w96) -> ()
                  }
                  frame Error {
                    n211 = One Button Dialog(message="手臂異常") -> ()  [unwired: 1 in, 1 out]
                    n212 = local write "StartCalib"(FALSE ("StartCalib")) -> ()
                  }
                }
              }
            }
          }
          frame "Snap" {
            n213 = call "ImgCtrl.vi"("Action"=enum16{"Initial", "read", "release"}."read", "ColorImg"=ColorImg."CBShow") -> ("ColorImg"=w109:string)  [unwired: 8 in, 1 out]
            n214 = call "ImgCtrl.vi"("Action"=enum16{"Initial", "read", "release"}."read", "ColorImg"=ColorImg."CBSource") -> ("ColorImg"=w106:string)  [unwired: 8 in, 1 out]
            n215 = call "IMAQ Copy"("Image Dst"=w109, "Image Src"=w106) -> ("error out"=w103:errorcluster, "Image Dst Out"=w110:T3)  [unwired: 4 in]
            n216 = local write "CalibBoardImg"(w110) -> ()
            n217 = case shown="No Error" w103 {
              frame No Error {
                n218 = local read "StartCalib"() -> (w111:bool)
                n219 = case shown="True" w111 {
                  frame False {
                  }
                  frame True {
                    n220 = local read "ActQ"() -> (w113:refnum<queue>)
                    n221 = Enqueue Element(queue=w113, element=CalibBoardAction."BoardCircleDectect") -> ()  [unwired: 2 in, 3 out]
                  }
                }
              }
              frame Error {
              }
            }
          }
          frame "BoardCircleDectect" {
            n222 = local read "Clu_BoardCircleParameter"() -> (w126:T5)
            n223 = local read "Circle Descriptor"() -> (w127:cluster{"Min Radius":dbl, "Max Radius":dbl})
            n224 = call "ImgCtrl.vi"("Action"=enum16{"Initial", "read", "release"}."read", "ColorImg"=ColorImg."CBToProcess") -> ("ColorImg"=w121:string)  [unwired: 8 in, 1 out]
            n225 = call "ImgCtrl.vi"("Action"=enum16{"Initial", "read", "release"}."read", "ColorImg"=ColorImg."CBShow") -> ("ColorImg"=w116:string)  [unwired: 8 in, 1 out]
            n226 = local read "ROI"() -> (w132:T6)
            n227 = Unbundle(w126) -> ("Extraction Mode"=w125:enum16{"Normal", "Uniform Regions"}, "Edge Threshold"=w124:i32, "Edge Filter Size"=w123:enum16{"Fine", "Normal"})
            n228 = call "IMAQ Copy"("Image Dst"=w121, "Image Src"=w116) -> ("Image Dst Out"=w122:T3)  [unwired: 4 in, 1 out]
            n229 = Unbundle(w132) -> ("left"=w133:i32, "Top"=w134:i32, "right"=w135:i32, "bottom"=w136:i32)
            n230 = Bundle By Name(cluster=T11 {"Curve Parameters"={"Extraction Mode"=enum."Normal", "Edge Threshold"=75, "Edge Filter Size"=enum."Normal", "Min Length"=25, "Row Search Step Size"=15, "Col Search Step Size"=15, "Max Endpoint Gap"=10, "Closed"=FALSE, "Subpixel"=FALSE}, "Circle Descriptor"={"Min Radius"=3.0, "Max Radius"=500.0}, "Match Options"={"Rotation"=TRUE, "Scale"=FALSE, "Occlusion"=FALSE, "Range Settings"=[{"Match Constraints"=enum."Rotation Angle (degrees)", "Min"=0.0, "Max"=360.0}]}, "Minimum match score"=100.0, "SetCircleNum"=1} ("ParameterIn"), "Curve Parameters.Extraction Mode"=w125, "Curve Parameters.Edge Threshold"=w124, "Curve Parameters.Edge Filter Size"=w123, "Circle Descriptor"=w127) -> (w129:T11)
            n231 = Bundle("left"=w133, "Top"=w134, "right"=w135, "bottom"=w136, 0.0) -> (w137:T18)  [unwired: 1 in]
            n232 = call "IMAQ Convert Rectangle to ROI"("Rectangle"=w137) -> ("ROI Descriptor"=w131:T19)  [unwired: 8 in, 1 out]
            n233 = call "ShapeDetection Circle.vi"("Image Dst In"=w122, "ParameterIn"=w129, "ROI Descriptor"=w131) -> ("Image Out"=w130:T3, "Circles"=w139:T4, "Numbers"=w115:i32)  [unwired: 12 in, 2 out]
            "Numbers" <- w115
            n234 = local read "StartCalib"() -> (w114:bool)
            n235 = local write "CalibBoardImg"(w130) -> ()
            n236 = local write "CirclesResult"(w139) -> ()
            n237 = case shown="True" w114 {
              tunnel: w115 -> [_ w142]
              frame False {
              }
              frame True {
                n238 = Equal?(x=1, y=w142) -> (x = y?=w140:bool)
                n239 = case shown="True" w140 {
                  frame False {
                    n240 = local write "StartCalib"(FALSE ("StartCalib")) -> ()
                    n241 = One Button Dialog(message="檢測錯誤") -> ()  [unwired: 1 in, 1 out]
                  }
                  frame True {
                    n242 = local read "ActQ"() -> (w146:refnum<queue>)
                    n243 = Enqueue Element(queue=w146, element=CalibBoardAction."CaculateOffset") -> ()  [unwired: 2 in, 3 out]
                  }
                }
              }
            }
          }
          frame "CaculateOffset" {
            w161 = 2
            n244 = local read "CalibBoardImg"() -> (w155:T3)
            n245 = local read "CirclesResult"() -> (w156:T4)
            n246 = call "Imaq GetImageInfo"("Image"=w155) -> ("Y Resolution"=w162:i32, "X Resolution"=w163:i32)  [unwired: 3 in, 6 out]
            n247 = Divide(x=w162, y=w161) -> (x/y=w159:dbl)
            n248 = Divide(x=w163, y=w161) -> (x/y=w160:dbl)
            n249 = Index Array(array=w156) -> (element=w165:T20)  [unwired: 1 in]
            n250 = Bundle(w160, w159) -> (w158:cluster{dbl, dbl})  [unwired: 1 in]
            n251 = Unbundle By Name(w165) -> ("Position"=w164:cluster{"X":sgl, "Y":sgl})
            n252 = global read "PanelSetting.vi" "UpScale"() -> (w154:dbl)
            n253 = Subtract(x=w164, y=w158) -> (x-y=w157:cluster{dbl, dbl})
            n254 = Multiply(x=w157, y=w154) -> (x*y=w147:cluster{dbl, dbl})
            n255 = Absolute Value(x=w147) -> (abs(x)=w153:cluster{dbl, dbl})
            n256 = Less Or Equal?(x=w153, y=15.0) -> (x <= y?=w151:cluster{bool, bool})
            n257 = Unbundle(w151) -> (w150:bool, w149:bool)
            n258 = And(x=w150, y=w149) -> (x .and. y?=w148:bool)
            n259 = case shown="True" w148 {
              tunnel: w147 -> [_ w174]
              frame False {
                n260 = One Button Dialog(message="檢測偏移過大") -> ()  [unwired: 1 in, 1 out]
              }
              frame True {
                n261 = Unbundle(w174) -> (w170:dbl, w168:dbl)
                n262 = Negate(x=w170) -> (-x=w169:dbl)
                n263 = Absolute Value(x=w169) -> (abs(x)=w184:dbl)
                n264 = Absolute Value(x=w168) -> (abs(x)=w181:dbl)
                n265 = call "Build Text2"("X"=w169, "Y"=w168) -> ("Result"=w175:string)  [unwired: 12 in, 1 out]
                n266 = Less Or Equal?(x=w184, y=0.01) -> (x <= y?=w179:bool)
                n267 = Less Or Equal?(x=w181, y=0.01) -> (x <= y?=w180:bool)
                n268 = And(x=w179, y=w180) -> (x .and. y?=w167:bool)
                n269 = call "SendPosToRobot.vi"("Timeout(ms)"=u32 2000, "PM"=T9 {"PM_1"=1, "PM_2"=1}, "Position"=w175, "RobotCmd"="RobotAction") -> ("error out"=w172:errorcluster, "position"=w173:string)  [unwired: 4 in, 2 out]
                n270 = call "FilterRobotPos.vi"("Cmd"=w173) -> ("Pos"=w171:dbl[])
                n271 = case shown="No Error" w172 {
                  tunnel: w171 -> [w186 _]
                  tunnel: w167 -> [w185 _]
                  frame No Error {
                    n272 = case shown="True" w185 {
                      tunnel: w186 -> [_ w208]
                      frame False {
                        n273 = stacked-sequence {
                          frame #0 {
                            n274 = Wait (ms)(milliseconds to wait=u32 300) -> ()  [unwired: 1 out]
                          }
                          frame #1 {
                            n275 = local read "ActQ"() -> (w189:refnum<queue>)
                            n276 = Enqueue Element(queue=w189, element=CalibBoardAction."Snap") -> ()  [unwired: 2 in, 3 out]
                          }
                        }
                      }
                      frame True {
                        n277 = To Single Precision Float(number=w208) -> (single precision float=w201:sgl[])
                        n278 = local read "UpCamTool"() -> (w200:refnum<vi>)
                        n279 = Index Array(array=w201) -> (element #1=w197:sgl, element #2=w195:sgl, element #3=w192:sgl, element #4=w191:sgl)  [unwired: 4 in]
                        n280 = property class="Clust (strict)"(reference=w200) -> ("Value"=w199:cluster{"CP-J1-X":sgl, "CP-J2-Y":sgl})  [unwired: 1 in, 2 out]
                        n281 = Unbundle(w199) -> ("CP-J1-X"=w198:sgl, "CP-J2-Y"=w196:sgl)
                        n282 = Add(x=w197, y=w198) -> (x+y=w194:sgl)
                        n283 = Add(x=w195, y=w196) -> (x+y=w193:sgl)
                        n284 = Build Array(w194, w193, w192, w191) -> (w190:sgl[])
                        n285 = local read "CalibPts"() -> (w205:cluster{"X":dbl, "Y":dbl, "Z":dbl, "U":dbl}[])
                        n286 = local read "Index"() -> (w207:i32)
                        n287 = Array To Cluster(array=w190) -> (cluster=w209:T21)
                        n288 = Decrement(x=w207) -> (x-1=w206:i32)
                        n289 = local read "ActQ"() -> (w203:refnum<queue>)
                        n290 = Replace Array Subset(array=w205, new element=w209, index=w206) -> (w204:cluster{"X":dbl, "Y":dbl, "Z":dbl, "U":dbl}[])
                        n291 = local write "CalibPts"(w204) -> ()
                        n292 = Enqueue Element(queue=w203, element=CalibBoardAction."CalibBoard") -> ()  [unwired: 2 in, 3 out]
                      }
                    }
                  }
                  frame Error {
                    n293 = local write "StartCalib"(FALSE ("StartCalib")) -> ()
                    n294 = One Button Dialog(message="手臂異常") -> ()  [unwired: 1 in, 1 out]
                  }
                }
              }
            }
          }
          frame "Exit" {
          }
        }
      }
      n295 = stacked-sequence {
        tunnel: w45 -> [_]
        frame #0 {
          n296 = local read "ActQ"() -> (w49:refnum<queue>)
          n297 = Enqueue Element(queue=w49, element=CalibBoardAction."Exit") -> ()  [unwired: 2 in, 3 out]
        }
      }
    }
  }
